vi "Set Averaging Period.vi"(8 "error in (no error)":errorcluster, 9 "Period (0.1s to 1s)":dbl=1.0 min=0.1 max=1.0, 11 "EPU452 in":refnum<class "EPU452.lvclass">) -> (0 "error out":errorcluster, 2 "Response":string, 3 "EPU452 out":refnum<class "EPU452.lvclass">)   [LabVIEW 2018, in "EPU452.lvclass"]
uses:
  EPU452.lvclass
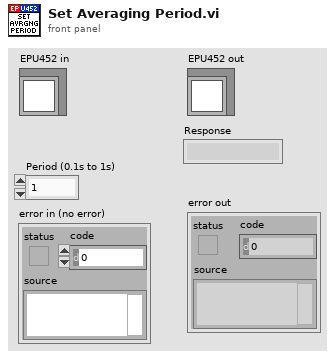
[diagram p1: front panel]
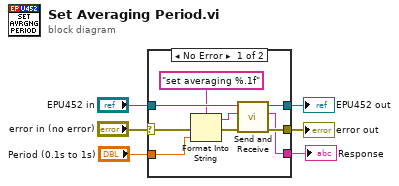
[diagram p0: block diagram]
diagram:
  n1 = case shown="No Error" "error in (no error)" {
    selector: "error in (no error)" -> [w14 w17]
    tunnel: [w13 w17] -> w5
    tunnel: [w12 w16] -> w3
    tunnel: "EPU452 in" -> [w15 w16]
    tunnel: "Period (0.1s to 1s)" -> [w11 _]
    tunnel: [w7 _] -> w1
    frame No Error {
      n2 = Format Into String(format string="set averaging %.1f", error in=w14, w11) -> (resulting string=w9:string, error out=w10:errorcluster)  [unwired: 1 in]
      n3 = call "Send and Receive.vi"("error in (no error)"=w10, "Command"=w9, "EPU452 in"=w15) -> ("error out"=w13:errorcluster, "Response"=w7:string, "EPU452 out"=w12:refnum<class "EPU452.lvclass">)  [unwired: 6 in]
    }
    frame Error {
    }
  }
  "error out" <- w5
  "EPU452 out" <- w3
  "Response" <- w1
